vi "csv_decomp.vi"(5 "Archivo de referencias (.csv)":path) -> (0 "finales":dbl[][](array[numeric]), 1 "iniciales":dbl[][](array[numeric]), 2 "etiquetas":string[][](array[string]), 3 "# dimención":i32, 7 "Lectura CSV":string[][](array[string]))   [LabVIEW 2017]
uses:
  <vilib>/Utility/file.llb/Read Delimited Spreadsheet (DBL).vi
  <vilib>/Utility/file.llb/Read Delimited Spreadsheet (string).vi
panel:
  out "Sample\ninicial":dbl[][](array[numeric])
  out "Sample\nfinal":dbl[][](array[numeric])
  out "Clase":string[][](array[string])
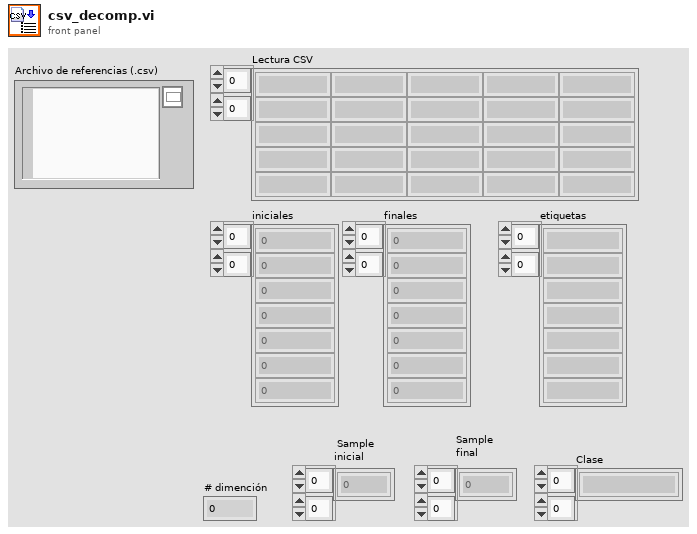
[diagram p1: front panel]
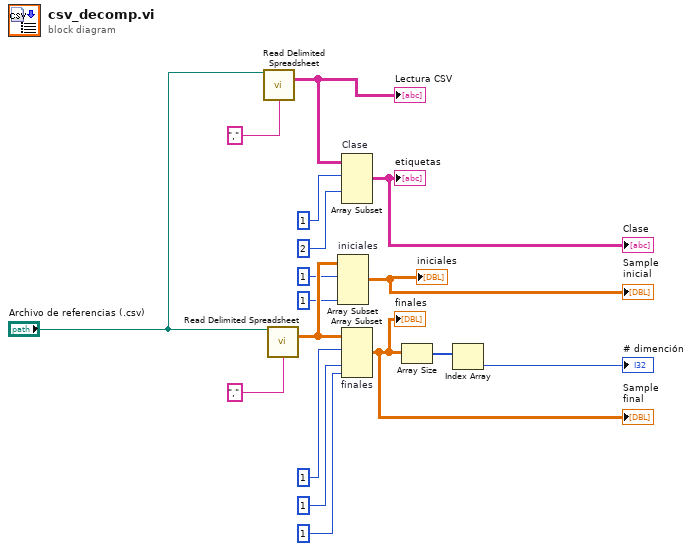
[diagram p0: block diagram]
diagram:
  n1 = call-poly <vilib>:"Read Delimited Spreadsheet.vi"("file path (dialog if empty)"="Archivo de referencias (.csv)", "delimiter (\\t)"="," ("delimiter (\\t)")) -> ("all rows"=w1:string[][])  [unwired: 8 in, 5 out]
  "Lectura CSV" <- w1
  n2 = call-poly <vilib>:"Read Delimited Spreadsheet.vi"("file path (dialog if empty)"="Archivo de referencias (.csv)", "delimiter (\\t)"="," ("delimiter (\\t)")) -> ("all rows"=w5:dbl[][])  [unwired: 8 in, 5 out]
  n3 = Array Subset "iniciales"(array=w5, index (row)=1 ("index"), length (col)=1 ("length")) -> (→"iniciales" →"Sample\ninicial":dbl[][])  [unwired: 2 in]
  n4 = Array Subset "Clase"(array=w1, index (row)=1 ("index"), index (col)=2 ("index")) -> (→"etiquetas" →"Clase":string[][])  [unwired: 2 in]
  n5 = Array Subset "finales"(array=w5, index (row)=1 ("index"), index (col)=1 ("index"), length (col)=1 ("length")) -> (w12:dbl[][])  [unwired: 1 in]
  "finales" <- w12
  "Sample\nfinal" <- w12
  n6 = Array Size(array=w12) -> (size(s)=w9:i32[])
  n7 = Index Array(array=w9) -> (element=→"# dimención":i32)  [unwired: 1 in]
